vi "PCP ype to max range.vi"(7 "PCP/PSU range":T1) -> (8 "Scale.Range:Maximum":dbl)   [LabVIEW 2011]
uses:
  PCP type List.ctl
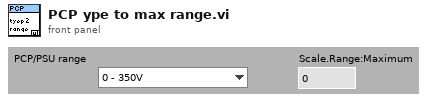
[diagram p1: front panel]
types:
  T1 = typedef "PCP type List.ctl" = enum16{"0 - 350V", "0 - 450V", "0 - 600V"}
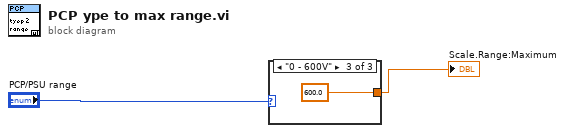
[diagram p0: block diagram]
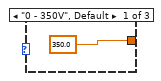
[diagram p2: hidden frame]
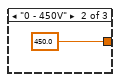
[diagram p3: hidden frame]
diagram:
  n1 = case shown="\"0 - 600V\"" "PCP/PSU range" {
    tunnel: [350.0 ("Scale.Range:Maximum") 450.0 ("Scale.Range:Maximum") 600.0 ("Scale.Range:Maximum")] -> w2
    frame "0 - 350V", Default {
    }
    frame "0 - 450V" {
    }
    frame "0 - 600V" {
    }
  }
  "Scale.Range:Maximum" <- w2
